vi "Main.vi"() -> ()   [LabVIEW 2014, in "Main Libraryv2.lvlib"]
uses:
  Control/Main Libraryv2.lvlib
  Master/Masterv2.lvclass
  Global/Recipe downloadv2.vi
  Global/Clockwise.Reverse Global.vi
  Global/Admin Enable Globalv2.vi
  Global/User Enablev2.vi
panel:
  in  "Login":bool
  out "Elapsed Time (s)":dbl
  out "Time has Elapsed":bool
  out "error out":errorcluster
  in  "error in (no error)":errorcluster
  out "User Enable":bool
  out "Admin Enable":bool
  in  "Log Out":bool
  in  "Tab Control 2":T1(tab)
  out "Direction":string
  out "Time Limit 2":string
  out "Temperature Limit 2":string
  out "Speed 2":string
  out "Timer":u16
  out "Current Temperature":u16
  in  "Delete":bool
  in  "Add":bool
  in  "Password List":i32(listbox)
  in  "New Password":string
  in  "Recipe Download":u16
  in  "Speed":u16
  in  "Time Limit":u16
  in  "Temperature Limit":u16
  in  "Delete Row":u16
  in  "Recipe":i32(listbox)
  in  "Delete Recipe":bool
  in  "Add Recipe":bool
  in  "Clockwise/Reverse":bool
  in  "Password List 2":i32(listbox)
  in  "Admin Password":string
  in  "Add Admin":bool
  in  "Delete Admin":bool
  in  "Pre Heat and Dry":bool
  in  "Exit":bool
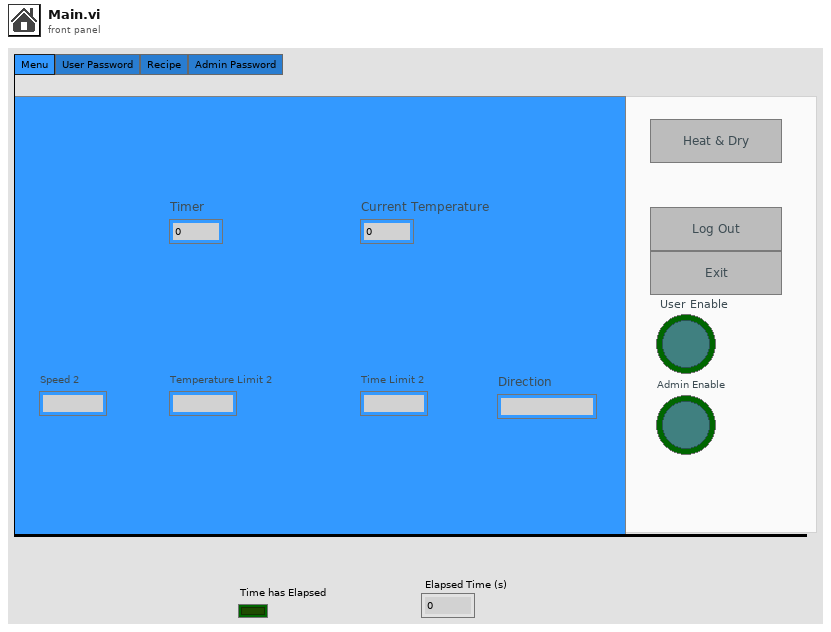
[diagram p1: front panel]
types:
  T1 = enum32{"Menu", "User Password", "Recipe", "Admin Password"}
  T2 = enum16{"9", "8", "7", "6", "5", "4", "3", "2", "1", "0"}[]
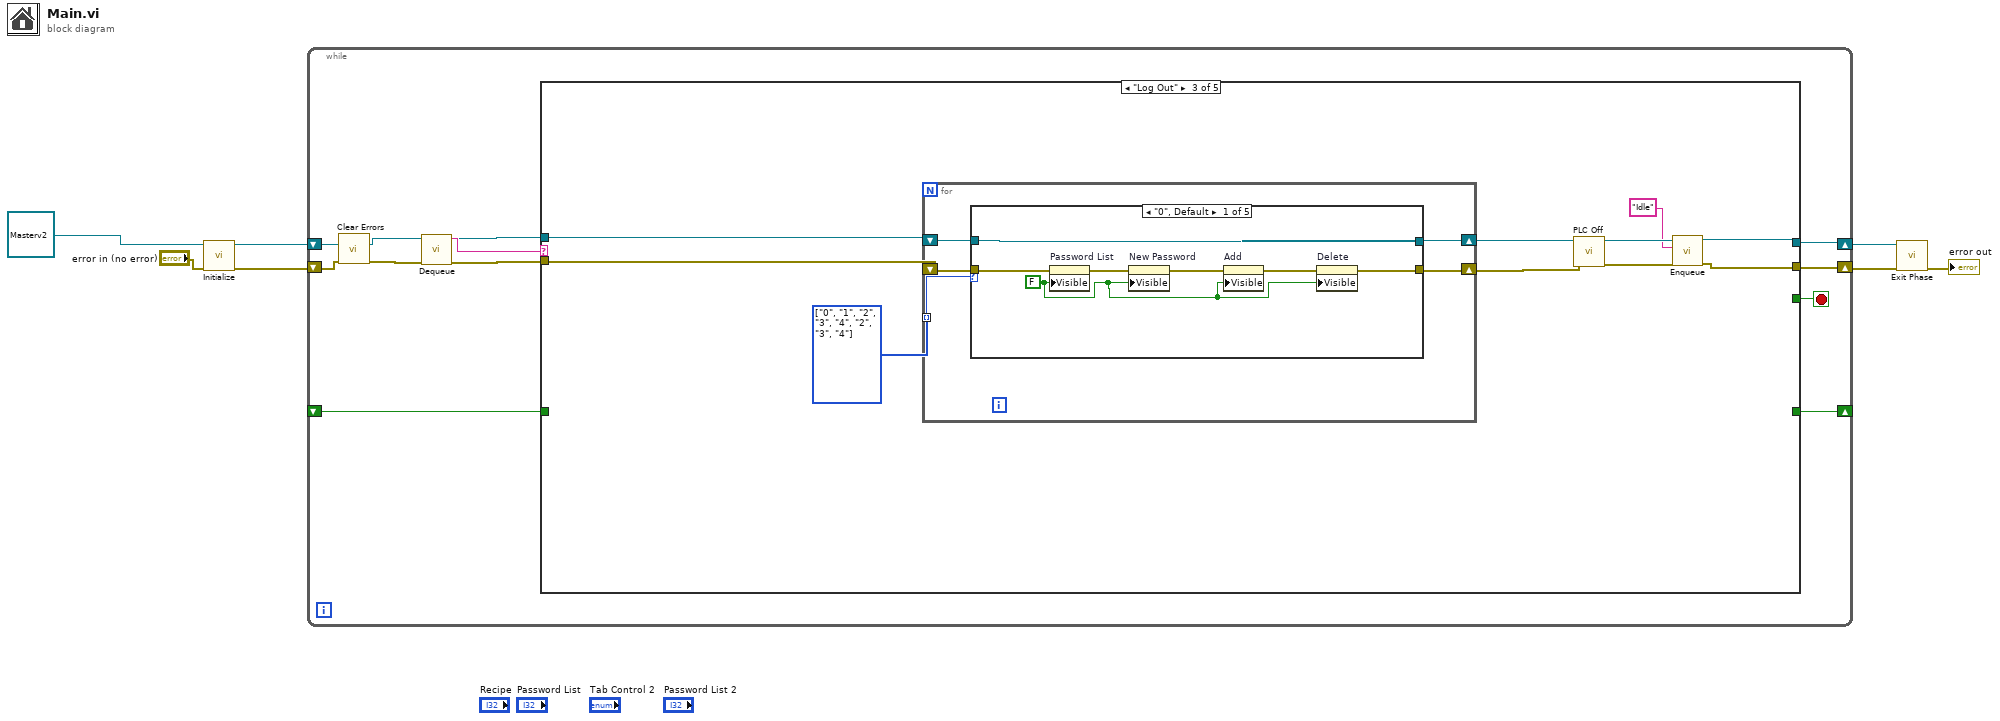
[diagram p0: block diagram]
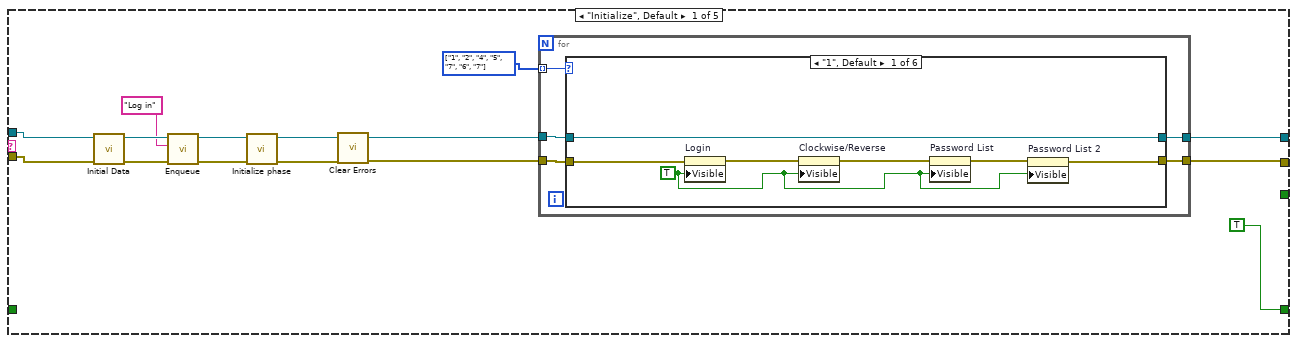
[diagram p2: hidden frame]
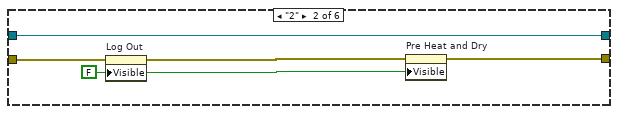
[diagram p3: hidden frame]
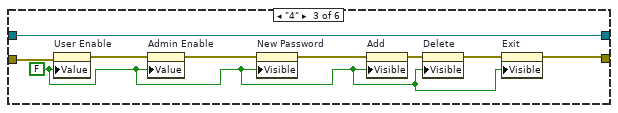
[diagram p4: hidden frame]
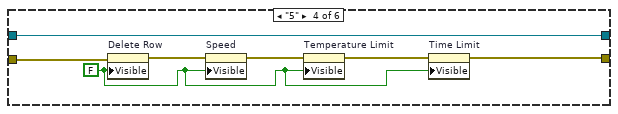
[diagram p5: hidden frame]
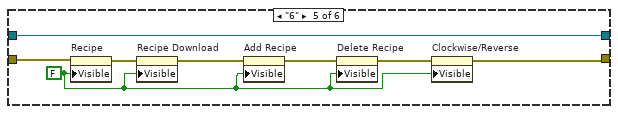
[diagram p6: hidden frame]
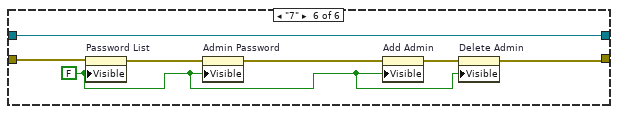
[diagram p7: hidden frame]
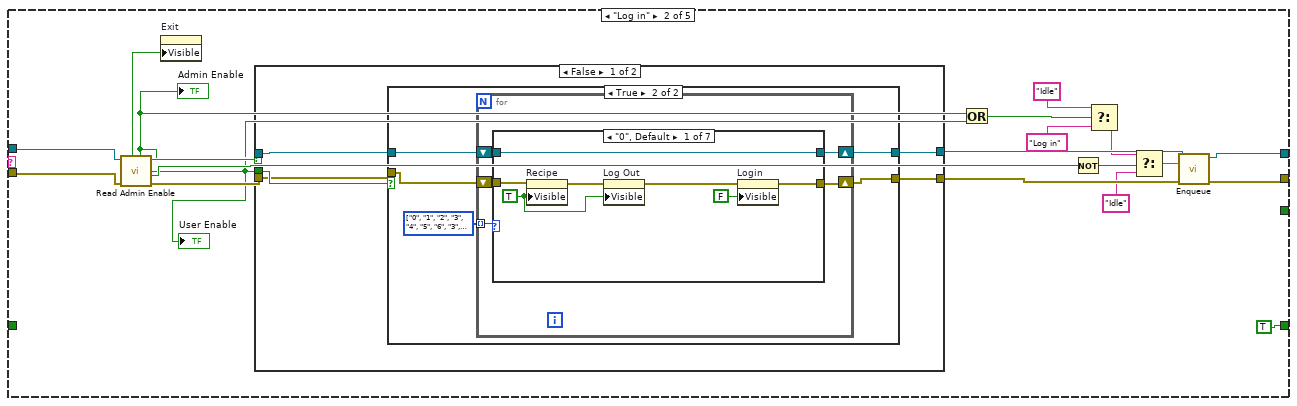
[diagram p8: hidden frame]
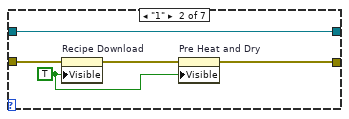
[diagram p10: hidden frame]
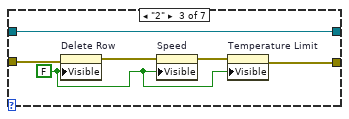
[diagram p11: hidden frame]
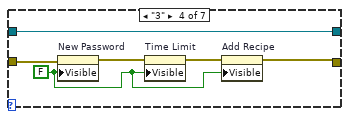
[diagram p12: hidden frame]
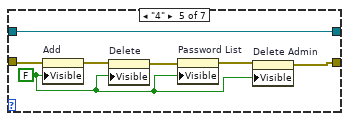
[diagram p13: hidden frame]
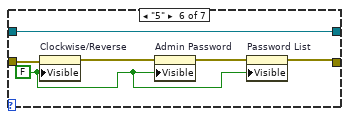
[diagram p14: hidden frame]
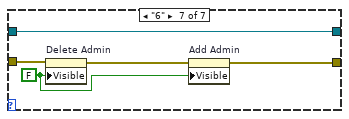
[diagram p15: hidden frame]
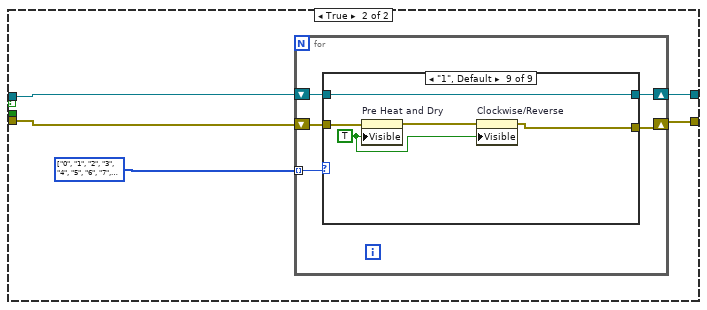
[diagram p16: hidden frame]
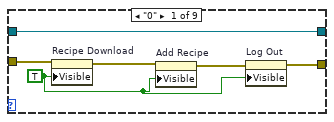
[diagram p17: hidden frame]
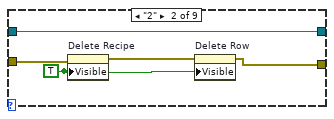
[diagram p18: hidden frame]
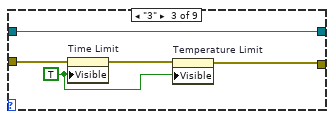
[diagram p19: hidden frame]
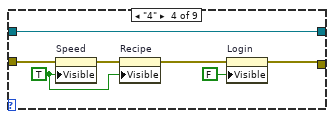
[diagram p20: hidden frame]
diagram:
  n1 = call-dynamic "Initialize.vi"("error in (no error)"="error in (no error)", "Masterv2 in"=refnum<class "Masterv2.lvclass"> refnum ("Main Library.lvlib:Masterv2.lvclass")) -> ("error out"=w4:errorcluster, "Masterv2 out"=w5:refnum<class "Masterv2.lvclass">)  [unwired: 8 in]
  n2 = while {
    shift-right: [w8] -> w2
    shift-left: w4 -> [w18]
    shift-right: [w10] -> w3
    shift-left: w5 -> [w16]
    shift-right: [w12] -> _
    shift-left: _ -> [w11]
    stop <- w9 stop-if-true
    n3 = call <vilib>:"Clear Errors.vi"("error in (no error)"=w18) -> ("error out"=w17:errorcluster)  [unwired: 5 in, 1 out]
    n4 = call-dynamic "Dequeue.vi"("error in (no error)"=w17, "Masterv2 in"=w16) -> ("error out"=w13:errorcluster, "Masterv2 out"=w14:refnum<class "Masterv2.lvclass">, "state"=w15:string)  [unwired: 7 in]
    n5 = case shown="\"Log Out\"" w15 {
      tunnel: w14 -> [w31 w95 w229 w276 w633]
      tunnel: w13 -> [w32 w94 w228 w275 w632]
      tunnel: [TRUE TRUE _ w273 _] -> w12
      tunnel: w11 -> [_ _ _ w274 _]
      tunnel: [w20 w92 w223 w272 w631] -> w10
      tunnel: [w19 w81 w221 w271 w629] -> w8
      tunnel: [_ _ _ _ TRUE] -> w9
      frame "Initialize", Default {
        w23 = enum16{"6", "7", "5", "4", "1", "2"}[] [enum."1", enum."2", enum."4", enum."5", enum."7", enum."6", enum."7"] items=["6", "7", "5", "4", "1", "2"]
        n6 = call-dynamic "Initial Data.vi"("error in (no error)"=w32, "Masterv2 in"=w31) -> ("error out"=w27:errorcluster, "Masterv2 out"=w30:refnum<class "Masterv2.lvclass">)  [unwired: 8 in]
        n7 = call-dynamic "Enqueue.vi"("error in (no error)"=w27, "State"="Log in", "Masterv2 in"=w30) -> ("error out"=w26:errorcluster, "Masterv2 out"=w28:refnum<class "Masterv2.lvclass">)  [unwired: 7 in]
        n8 = call-dynamic "Initialize phase.vi"("error in (no error)"=w26, "Programming Logicv2 in"=w28) -> ("error out"=w25:errorcluster, "Programming Logicv2 out"=w21:refnum<class "Masterv2.lvclass">)  [unwired: 8 in]
        n9 = call <vilib>:"Clear Errors.vi"("error in (no error)"=w25) -> ("error out"=w22:errorcluster)  [unwired: 5 in, 1 out]
        n10 = for {
          tunnel: w23 -> [w37] mode=indexing
          tunnel: w21 -> [w36]
          tunnel: [w35] -> w20
          tunnel: w22 -> [w34]
          tunnel: [w33] -> w19
          n11 = case shown="\"1\", Default" w37 {
            tunnel: w36 -> [w44 w49 w58 w65 w73 w80]
            tunnel: [w44 w49 w58 w65 w73 w80] -> w35
            tunnel: w34 -> [w43 w48 w57 w64 w72 w79]
            tunnel: [w38 w46 w51 w60 w67 w75] -> w33
            frame "1", Default {
              w39 = TRUE ("Visible")
              n12 = property on="Login" class="Bool"(error in=w43, "Visible"=w39) -> (error out=w42:errorcluster)  [unwired: 1 in, 1 out]
              n13 = property on="Clockwise/Reverse" class="Bool (strict)"(error in=w42, "Visible"=w39) -> (error out=w41:errorcluster)  [unwired: 1 in, 1 out]
              n14 = property on="Password List" class="LstBox (strict)"(error in=w41, "Visible"=w39) -> (error out=w40:errorcluster)  [unwired: 1 in, 1 out]
              n15 = property on="Password List 2" class="LstBox (strict)"(error in=w40, "Visible"=w39) -> (error out=w38:errorcluster)  [unwired: 1 in, 1 out]
            }
            frame "2" {
              w45 = FALSE ("Visible")
              n16 = property on="Log Out" class="Bool (strict)"(error in=w48, "Visible"=w45) -> (error out=w47:errorcluster)  [unwired: 1 in, 1 out]
              n17 = property on="Pre Heat and Dry" class="Bool (strict)"(error in=w47, "Visible"=w45) -> (error out=w46:errorcluster)  [unwired: 1 in, 1 out]
            }
            frame "4" {
              w50 = FALSE ("User Enable")
              n18 = property on="User Enable" class="Bool (strict)"(error in=w57, "Value"=w50) -> (error out=w56:errorcluster)  [unwired: 1 in, 1 out]
              n19 = property on="Admin Enable" class="Bool (strict)"(error in=w56, "Value"=w50) -> (error out=w55:errorcluster)  [unwired: 1 in, 1 out]
              n20 = property on="New Password" class="Str"(error in=w55, "Visible"=w50) -> (error out=w54:errorcluster)  [unwired: 1 in, 1 out]
              n21 = property on="Add" class="Bool"(error in=w54, "Visible"=w50) -> (error out=w53:errorcluster)  [unwired: 1 in, 1 out]
              n22 = property on="Delete" class="Bool"(error in=w53, "Visible"=w50) -> (error out=w52:errorcluster)  [unwired: 1 in, 1 out]
              n23 = property on="Exit" class="Bool"(error in=w52, "Visible"=w50) -> (error out=w51:errorcluster)  [unwired: 1 in, 1 out]
            }
            frame "5" {
              w59 = FALSE ("Visible")
              n24 = property on="Delete Row" class="DigNum (strict)"(error in=w64, "Visible"=w59) -> (error out=w63:errorcluster)  [unwired: 1 in, 1 out]
              n25 = property on="Speed" class="DigNum (strict)"(error in=w63, "Visible"=w59) -> (error out=w62:errorcluster)  [unwired: 1 in, 1 out]
              n26 = property on="Temperature Limit" class="DigNum (strict)"(error in=w62, "Visible"=w59) -> (error out=w61:errorcluster)  [unwired: 1 in, 1 out]
              n27 = property on="Time Limit" class="DigNum (strict)"(error in=w61, "Visible"=w59) -> (error out=w60:errorcluster)  [unwired: 1 in, 1 out]
            }
            frame "6" {
              w66 = FALSE ("Visible")
              n28 = property on="Recipe" class="MCListbox (strict)"(error in=w72, "Visible"=w66) -> (error out=w71:errorcluster)  [unwired: 1 in, 1 out]
              n29 = property on="Recipe Download" class="DigNum (strict)"(error in=w71, "Visible"=w66) -> (error out=w70:errorcluster)  [unwired: 1 in, 1 out]
              n30 = property on="Add Recipe" class="Bool"(error in=w70, "Visible"=w66) -> (error out=w69:errorcluster)  [unwired: 1 in, 1 out]
              n31 = property on="Delete Recipe" class="Bool"(error in=w69, "Visible"=w66) -> (error out=w68:errorcluster)  [unwired: 1 in, 1 out]
              n32 = property on="Clockwise/Reverse" class="Bool (strict)"(error in=w68, "Visible"=w66) -> (error out=w67:errorcluster)  [unwired: 1 in, 1 out]
            }
            frame "7" {
              w74 = FALSE ("Visible")
              n33 = property on="Password List" class="LstBox (strict)"(error in=w79, "Visible"=w74) -> (error out=w78:errorcluster)  [unwired: 1 in, 1 out]
              n34 = property on="Admin Password" class="Str"(error in=w78, "Visible"=w74) -> (error out=w77:errorcluster)  [unwired: 1 in, 1 out]
              n35 = property on="Add Admin" class="Bool"(error in=w77, "Visible"=w74) -> (error out=w76:errorcluster)  [unwired: 1 in, 1 out]
              n36 = property on="Delete Admin" class="Bool"(error in=w76, "Visible"=w74) -> (error out=w75:errorcluster)  [unwired: 1 in, 1 out]
            }
          }
        }
      }
      frame "Log in" {
        n37 = call-dynamic "Read Admin Enable.vi"("error in (no error)"=w94, "Masterv2 in"=w95) -> ("error out"=w96:errorcluster, "Boolean"=w84:bool, "Masterv2 out"=w97:refnum<class "Masterv2.lvclass">, "Admin Enable"=w83:bool, "User Enable"=w82:bool, "Programmer Enable"=w93:bool)  [unwired: 4 in]
        "Admin Enable" <- w83
        "User Enable" <- w82
        n38 = property on="Exit" class="Bool"("Visible"=w93) -> ()  [unwired: 2 in, 2 out]
        n39 = case shown="False" w83 {
          tunnel: w82 -> [w105 _]
          tunnel: w96 -> [w103 w164]
          tunnel: w97 -> [w104 w162]
          tunnel: [w101 w163] -> w98
          tunnel: [w102 w161] -> w99
          frame False {
            n40 = case shown="True" w105 {
              tunnel: w104 -> [w107 w112]
              tunnel: w103 -> [w106 w111]
              tunnel: [w107 w110] -> w102
              tunnel: [w106 w109] -> w101
              frame False {
              }
              frame True {
                w108 = enum16{"6", "5", "4", "3", "2", "1", "0"}[] [enum."0", enum."1", enum."2", enum."3", enum."4", enum."5", enum."6", enum."3", enum."4", enum."5", enum."6"] items=["6", "5", "4", "3", "2", "1", "0"]
                n41 = for {
                  shift-right: [w115] -> w110
                  shift-left: w112 -> [w116]
                  shift-right: [w113] -> w109
                  shift-left: w111 -> [w117]
                  tunnel: w108 -> [w114] mode=indexing
                  n42 = case shown="\"0\", Default" w114 {
                    tunnel: w117 -> [w123 w128 w134 w140 w145 w153 w158]
                    tunnel: w116 -> [w124 w129 w135 w141 w148 w154 w159]
                    tunnel: [w124 w129 w135 w141 w148 w154 w159] -> w115
                    tunnel: [w120 w126 w131 w137 w143 w150 w156] -> w113
                    frame "0", Default {
                      w119 = TRUE ("Visible")
                      n43 = property on="Recipe" class="MCListbox (strict)"(error in=w123, "Visible"=w119) -> (error out=w122:errorcluster)  [unwired: 1 in, 1 out]
                      n44 = property on="Log Out" class="Bool (strict)"(error in=w122, "Visible"=w119) -> (error out=w121:errorcluster)  [unwired: 1 in, 1 out]
                      n45 = property on="Login" class="Bool"(error in=w121, "Visible"=FALSE) -> (error out=w120:errorcluster)  [unwired: 1 in, 1 out]
                    }
                    frame "1" {
                      w125 = TRUE ("Visible")
                      n46 = property on="Recipe Download" class="DigNum (strict)"(error in=w128, "Visible"=w125) -> (error out=w127:errorcluster)  [unwired: 1 in, 1 out]
                      n47 = property on="Pre Heat and Dry" class="Bool (strict)"(error in=w127, "Visible"=w125) -> (error out=w126:errorcluster)  [unwired: 1 in, 1 out]
                    }
                    frame "2" {
                      w130 = FALSE ("Visible")
                      n48 = property on="Delete Row" class="DigNum (strict)"(error in=w134, "Visible"=w130) -> (error out=w133:errorcluster)  [unwired: 1 in, 1 out]
                      n49 = property on="Speed" class="DigNum (strict)"(error in=w133, "Visible"=w130) -> (error out=w132:errorcluster)  [unwired: 1 in, 1 out]
                      n50 = property on="Temperature Limit" class="DigNum (strict)"(error in=w132, "Visible"=w130) -> (error out=w131:errorcluster)  [unwired: 1 in, 1 out]
                    }
                    frame "3" {
                      w136 = FALSE ("Visible")
                      n51 = property on="New Password" class="Str"(error in=w140, "Visible"=w136) -> (error out=w139:errorcluster)  [unwired: 1 in, 1 out]
                      n52 = property on="Time Limit" class="DigNum (strict)"(error in=w139, "Visible"=w136) -> (error out=w138:errorcluster)  [unwired: 1 in, 1 out]
                      n53 = property on="Add Recipe" class="Bool"(error in=w138, "Visible"=w136) -> (error out=w137:errorcluster)  [unwired: 1 in, 1 out]
                    }
                    frame "4" {
                      w142 = FALSE ("Visible")
                      n54 = property on="Add" class="Bool"(error in=w145, "Visible"=w142) -> (error out=w146:errorcluster)  [unwired: 1 in, 1 out]
                      n55 = property on="Delete" class="Bool"(error in=w146, "Visible"=w142) -> (error out=w147:errorcluster)  [unwired: 1 in, 1 out]
                      n56 = property on="Password List" class="LstBox (strict)"(error in=w147, "Visible"=w142) -> (error out=w144:errorcluster)  [unwired: 1 in, 1 out]
                      n57 = property on="Delete Admin" class="Bool"(error in=w144, "Visible"=w142) -> (error out=w143:errorcluster)  [unwired: 1 in, 1 out]
                    }
                    frame "5" {
                      w149 = FALSE ("Visible")
                      n58 = property on="Clockwise/Reverse" class="Bool (strict)"(error in=w153, "Visible"=w149) -> (error out=w152:errorcluster)  [unwired: 1 in, 1 out]
                      n59 = property on="Admin Password" class="Str"(error in=w152, "Visible"=w149) -> (error out=w151:errorcluster)  [unwired: 1 in, 1 out]
                      n60 = property on="Password List" class="LstBox (strict)"(error in=w151, "Visible"=w149) -> (error out=w150:errorcluster)  [unwired: 1 in, 1 out]
                    }
                    frame "6" {
                      w155 = FALSE ("Visible")
                      n61 = property on="Delete Admin" class="Bool"(error in=w158, "Visible"=w155) -> (error out=w157:errorcluster)  [unwired: 1 in, 1 out]
                      n62 = property on="Add Admin" class="Bool"(error in=w157, "Visible"=w155) -> (error out=w156:errorcluster)  [unwired: 1 in, 1 out]
                    }
                  }
                }
              }
            }
          }
          frame True {
            w160 = T2 [enum."0", enum."1", enum."2", enum."3", enum."4", enum."5", enum."6", enum."7", enum."8", enum."9"] items=["9", "8", "7", "6", "5", "4", "3", "2", "1", "0"]
            n63 = for {
              shift-right: [w167] -> w161
              shift-left: w162 -> [w168]
              shift-right: [w165] -> w163
              shift-left: w164 -> [w169]
              tunnel: w160 -> [w166] mode=indexing
              n64 = case shown="\"1\", Default" w166 {
                tunnel: w169 -> [w174 w179 w184 w191 w197 w202 w207 w214 w219]
                tunnel: w168 -> [w175 w180 w185 w192 w198 w203 w208 w215 w220]
                tunnel: [w175 w180 w185 w192 w198 w203 w208 w215 w220] -> w167
                tunnel: [w171 w177 w182 w188 w193 w200 w205 w211 w217] -> w165
                frame "0" {
                  w170 = TRUE ("Visible")
                  n65 = property on="Recipe Download" class="DigNum (strict)"(error in=w174, "Visible"=w170) -> (error out=w173:errorcluster)  [unwired: 1 in, 1 out]
                  n66 = property on="Add Recipe" class="Bool"(error in=w173, "Visible"=w170) -> (error out=w172:errorcluster)  [unwired: 1 in, 1 out]
                  n67 = property on="Log Out" class="Bool (strict)"(error in=w172, "Visible"=w170) -> (error out=w171:errorcluster)  [unwired: 1 in, 1 out]
                }
                frame "2" {
                  w176 = TRUE ("Visible")
                  n68 = property on="Delete Recipe" class="Bool"(error in=w179, "Visible"=w176) -> (error out=w178:errorcluster)  [unwired: 1 in, 1 out]
                  n69 = property on="Delete Row" class="DigNum (strict)"(error in=w178, "Visible"=w176) -> (error out=w177:errorcluster)  [unwired: 1 in, 1 out]
                }
                frame "3" {
                  w181 = TRUE ("Visible")
                  n70 = property on="Time Limit" class="DigNum (strict)"(error in=w184, "Visible"=w181) -> (error out=w183:errorcluster)  [unwired: 1 in, 1 out]
                  n71 = property on="Temperature Limit" class="DigNum (strict)"(error in=w183, "Visible"=w181) -> (error out=w182:errorcluster)  [unwired: 1 in, 1 out]
                }
                frame "4" {
                  w187 = TRUE ("Visible")
                  n72 = property on="Speed" class="DigNum (strict)"(error in=w191, "Visible"=w187) -> (error out=w190:errorcluster)  [unwired: 1 in, 1 out]
                  n73 = property on="Recipe" class="MCListbox (strict)"(error in=w190, "Visible"=w187) -> (error out=w189:errorcluster)  [unwired: 1 in, 1 out]
                  n74 = property on="Login" class="Bool"(error in=w189, "Visible"=FALSE) -> (error out=w188:errorcluster)  [unwired: 1 in, 1 out]
                }
                frame "5" {
                  w194 = TRUE ("Visible")
                  n75 = property on="New Password" class="Str"(error in=w197, "Visible"=w194) -> (error out=w196:errorcluster)  [unwired: 1 in, 1 out]
                  n76 = property on="Delete" class="Bool"(error in=w196, "Visible"=w194) -> (error out=w195:errorcluster)  [unwired: 1 in, 1 out]
                  n77 = property on="Password List" class="LstBox (strict)"(error in=w195, "Visible"=w194) -> (error out=w193:errorcluster)  [unwired: 1 in, 1 out]
                }
                frame "6" {
                  w199 = TRUE ("Visible")
                  n78 = property on="Add" class="Bool"(error in=w202, "Visible"=w199) -> (error out=w201:errorcluster)  [unwired: 1 in, 1 out]
                  n79 = property on="Delete" class="Bool"(error in=w201, "Visible"=w199) -> (error out=w200:errorcluster)  [unwired: 1 in, 1 out]
                }
                frame "7" {
                  w204 = TRUE ("Visible")
                  n80 = property on="Password List" class="LstBox (strict)"(error in=w207, "Visible"=w204) -> (error out=w206:errorcluster)  [unwired: 1 in, 1 out]
                  n81 = property on="Admin Password" class="Str"(error in=w206, "Visible"=w204) -> (error out=w205:errorcluster)  [unwired: 1 in, 1 out]
                }
                frame "8" {
                  w210 = TRUE ("Visible")
                  n82 = property on="Add Admin" class="Bool"(error in=w214, "Visible"=w210) -> (error out=w213:errorcluster)  [unwired: 1 in, 1 out]
                  n83 = property on="Delete Admin" class="Bool"(error in=w213, "Visible"=w210) -> (error out=w212:errorcluster)  [unwired: 1 in, 1 out]
                  n84 = property on="Login" class="Bool"(error in=w212, "Visible"=FALSE) -> (error out=w211:errorcluster)  [unwired: 1 in, 1 out]
                }
                frame "1", Default {
                  w216 = TRUE ("Visible")
                  n85 = property on="Pre Heat and Dry" class="Bool (strict)"(error in=w219, "Visible"=w216) -> (error out=w218:errorcluster)  [unwired: 1 in, 1 out]
                  n86 = property on="Clockwise/Reverse" class="Bool (strict)"(error in=w218, "Visible"=w216) -> (error out=w217:errorcluster)  [unwired: 1 in, 1 out]
                }
              }
            }
          }
        }
        n87 = Or(x=w83, y=w82) -> (x .or. y?=w89:bool)
        n88 = Not(x=w84) -> (.not. x?=w87:bool)
        n89 = Select(t="Idle", s=w89, f="Log in" ("State")) -> (s? t:f=w88:string)
        n90 = Select(t=w88, s=w87, f="Idle") -> (s? t:f=w85:string)
        n91 = call-dynamic "Enqueue.vi"("error in (no error)"=w98, "State"=w85, "Masterv2 in"=w99) -> ("error out"=w81:errorcluster, "Masterv2 out"=w92:refnum<class "Masterv2.lvclass">)  [unwired: 7 in]
      }
      frame "Log Out" {
        w230 = enum16{"4", "3", "2", "1", "0"}[] [enum."0", enum."1", enum."2", enum."3", enum."4", enum."2", enum."3", enum."4"] items=["4", "3", "2", "1", "0"]
        n92 = for {
          shift-right: [w233] -> w225
          shift-left: w229 -> [w234]
          shift-right: [w231] -> w224
          shift-left: w228 -> [w232]
          tunnel: w230 -> [w235] mode=indexing
          n93 = case shown="\"0\", Default" w235 {
            tunnel: w234 -> [w242 w249 w257 w263 w270]
            tunnel: [w242 w249 w257 w263 w270] -> w233
            tunnel: w232 -> [w241 w248 w256 w262 w269]
            tunnel: [w237 w244 w252 w259 w265] -> w231
            frame "0", Default {
              w236 = FALSE ("Visible")
              n94 = property on="Password List" class="LstBox (strict)"(error in=w241, "Visible"=w236) -> (error out=w240:errorcluster)  [unwired: 1 in, 1 out]
              n95 = property on="New Password" class="Str"(error in=w240, "Visible"=w236) -> (error out=w239:errorcluster)  [unwired: 1 in, 1 out]
              n96 = property on="Add" class="Bool"(error in=w239, "Visible"=w236) -> (error out=w238:errorcluster)  [unwired: 1 in, 1 out]
              n97 = property on="Delete" class="Bool"(error in=w238, "Visible"=w236) -> (error out=w237:errorcluster)  [unwired: 1 in, 1 out]
            }
            frame "1" {
              w243 = FALSE ("Visible")
              n98 = property on="Recipe" class="MCListbox (strict)"(error in=w248, "Visible"=w243) -> (error out=w247:errorcluster)  [unwired: 1 in, 1 out]
              n99 = property on="Recipe Download" class="DigNum (strict)"(error in=w247, "Visible"=w243) -> (error out=w246:errorcluster)  [unwired: 1 in, 1 out]
              n100 = property on="Delete Row" class="DigNum (strict)"(error in=w246, "Visible"=w243) -> (error out=w245:errorcluster)  [unwired: 1 in, 1 out]
              n101 = property on="Log Out" class="Bool (strict)"(error in=w245, "Visible"=w243) -> (error out=w244:errorcluster)  [unwired: 1 in, 1 out]
            }
            frame "2" {
              w250 = FALSE ("Visible")
              n102 = property on="Speed" class="DigNum (strict)"(error in=w256, "Visible"=w250) -> (error out=w255:errorcluster)  [unwired: 1 in, 1 out]
              n103 = property on="Temperature Limit" class="DigNum (strict)"(error in=w255, "Visible"=w250) -> (error out=w254:errorcluster)  [unwired: 1 in, 1 out]
              n104 = property on="Time Limit" class="DigNum (strict)"(error in=w254, "Visible"=w250) -> (error out=w253:errorcluster)  [unwired: 1 in, 1 out]
              n105 = property on="Login" class="Bool"(error in=w253, "Visible"=TRUE) -> (error out=w252:errorcluster)  [unwired: 1 in, 1 out]
            }
            frame "3" {
              w258 = FALSE ("Visible")
              n106 = property on="Add Recipe" class="Bool"(error in=w262, "Visible"=w258) -> (error out=w261:errorcluster)  [unwired: 1 in, 1 out]
              n107 = property on="Delete Recipe" class="Bool"(error in=w261, "Visible"=w258) -> (error out=w260:errorcluster)  [unwired: 1 in, 1 out]
              n108 = property on="Clockwise/Reverse" class="Bool (strict)"(error in=w260, "Visible"=w258) -> (error out=w259:errorcluster)  [unwired: 1 in, 1 out]
            }
            frame "4" {
              w264 = FALSE ("Visible")
              n109 = property on="Password List" class="LstBox (strict)"(error in=w269, "Visible"=w264) -> (error out=w268:errorcluster)  [unwired: 1 in, 1 out]
              n110 = property on="Admin Password" class="Str"(error in=w268, "Visible"=w264) -> (error out=w267:errorcluster)  [unwired: 1 in, 1 out]
              n111 = property on="Add Admin" class="Bool"(error in=w267, "Visible"=w264) -> (error out=w266:errorcluster)  [unwired: 1 in, 1 out]
              n112 = property on="Delete Admin" class="Bool"(error in=w266, "Visible"=w264) -> (error out=w265:errorcluster)  [unwired: 1 in, 1 out]
            }
          }
        }
        n113 = call-dynamic "PLC Off.vi"("error in (no error)"=w224, "Programming Logicv2 in"=w225) -> ("error out"=w226:errorcluster, "Programming Logicv2 out"=w227:refnum<class "Masterv2.lvclass">)  [unwired: 8 in]
        n114 = call-dynamic "Enqueue.vi"("error in (no error)"=w226, "State"="Idle", "Masterv2 in"=w227) -> ("error out"=w221:errorcluster, "Masterv2 out"=w223:refnum<class "Masterv2.lvclass">)  [unwired: 7 in]
      }
      frame "Idle" {
        n115 = event shown="[0] Timeout" {
          selector: _ -> [_ _ _ _ _ _ _ _ _ _ _ _]
          dyn-events: _ -> [_ _ _ _ _ _ _ _ _ _ _ _]
          timeout: 100 -> [_ _ _ _ _ _ _ _ _ _ _ _]
          tunnel: w276 -> [w302 w313 w326 w459 w523 w537 w555 w569 w583 w597 w600 w617]
          tunnel: w275 -> [w301 w312 w327 w458 w522 w536 w554 w568 w582 w596 w604 w616]
          tunnel: w274 -> [w286 _ _ _ _ _ _ _ _ _ _ _]
          tunnel: [FALSE TRUE TRUE TRUE _ _ _ _ _ _ _ _] -> w273
          tunnel: [w283 w317 w330 w463 w513 w527 w545 w559 w573 w587 w610 w624] -> w272
          tunnel: [w282 w318 w329 w462 w512 w526 w544 w558 w572 w586 w609 w623] -> w271
          event Timeout {
            n116 = event-data() -> ()  [unwired: 1 in, 3 out]
            n117 = call-dynamic "Display Information.vi"("error in (no error)"=w301, "Masterv2 in"=w302) -> ("error out"=w294:errorcluster, "Passwords"=w299:string[], "Masterv2 out"=w295:refnum<class "Masterv2.lvclass">, "Recipe Indicator"=w298:string[][], "Passwords 2"=w300:string[])  [unwired: 5 in]
            n118 = property on="Password List 2" class="LstBox (strict)"("Item Names"=w300) -> ()  [unwired: 2 in, 2 out]
            n119 = property on="Password List" class="LstBox (strict)"("Item Names"=w299) -> ()  [unwired: 2 in, 2 out]
            n120 = property on="Recipe" class="MCListbox (strict)"("ItemNames"=w298) -> ()  [unwired: 2 in, 2 out]
            n121 = call-dynamic "Timeout Phase.vi"("error in (no error)"=w294, "Programming Logicv2 in"=w295) -> ("error out"=w293:errorcluster, "Boolean"=w285:bool, "Programming Logicv2 out"=w291:refnum<class "Masterv2.lvclass">, "Timer"=→"Timer":u16, "Temperature"=→"Current Temperature":u16)  [unwired: 5 in]
            n122 = Or(x=w285, y=w286) -> (x .or. y?=w287:bool)
            n123 = call <vilib>:"Clear Errors.vi"("error in (no error)"=w293) -> ("error out"=w292:errorcluster)  [unwired: 5 in, 1 out]
            n124 = call "Elapsed Time"("Time Target (s)"=600.0, "Reset"=w287, "Set Start Time (s)"=0.0) -> ("Elapsed Time (s)"=→"Elapsed Time (s)":dbl, "Time has Elapsed"=w278:bool)  [unwired: 9 in, 6 out]
            "Time has Elapsed" <- w278
            n125 = Select(t="Log Out", s=w278, f="Idle") -> (s? t:f=w279:string)
            n126 = call-dynamic "Enqueue.vi"("error in (no error)"=w292, "State"=w279, "Masterv2 in"=w291) -> ("error out"=w282:errorcluster, "Masterv2 out"=w283:refnum<class "Masterv2.lvclass">)  [unwired: 7 in]
          }
          event "Pre Heat and Dry": Mouse Up {
            n127 = event-data() -> ()  [unwired: 1 in, 8 out]
            n128 = property on="Recipe" class="MCListbox (strict)"() -> ("ItemNames"=w308:string[][])  [unwired: 2 in, 2 out]
            n129 = global write "Recipe downloadv2.vi" "Recipe Download"("Recipe Download") -> ()
            n130 = call-dynamic "Start Phase.vi"("array"=w308, "error in (no error)"=w312, "index (row)"="Recipe Download", "Programming Logicv2 in"=w313) -> ("error out"=w316:errorcluster, "Speed"=→"Speed 2":string, "Direction"=→"Direction":string, "Programming Logicv2 out"=w314:refnum<class "Masterv2.lvclass">, "Temp"=→"Temperature Limit 2":string, "Time"=→"Time Limit 2":string)  [unwired: 2 in]
            n131 = call <vilib>:"Clear Errors.vi"("error in (no error)"=w316) -> ("error out"=w315:errorcluster)  [unwired: 5 in, 1 out]
            n132 = global write "Clockwise.Reverse Global.vi" "Clockwise/Reverse"("Clockwise/Reverse") -> ()
            n133 = call-dynamic "Enqueue.vi"("error in (no error)"=w315, "State"="Idle", "Masterv2 in"=w314) -> ("error out"=w318:errorcluster, "Masterv2 out"=w317:refnum<class "Masterv2.lvclass">)  [unwired: 7 in]
          }
          event "Login": Value Change {
            n134 = event-data() -> ()  [unwired: 1 in, 6 out]
            n135 = call-dynamic "Read Admin Enable.vi"("error in (no error)"=w327, "Masterv2 in"=w326) -> ("error out"=w323:errorcluster, "Masterv2 out"=w324:refnum<class "Masterv2.lvclass">, "Admin Enable"=w321:bool, "User Enable"=w322:bool, "Programmer Enable"=w325:bool)  [unwired: 4 in, 1 out]
            n136 = property on="Exit" class="Bool"("Visible"=w325) -> ()  [unwired: 2 in, 2 out]
            n137 = global write "Admin Enable Globalv2.vi" "Admin Enable"(w321) -> ()
            n138 = global write "User Enablev2.vi" "User Enable"(w322) -> ()
            n139 = case shown="False" w321 {
              tunnel: w322 -> [w336 _]
              tunnel: w323 -> [w334 w397]
              tunnel: w324 -> [w335 w395]
              tunnel: [w332 w396] -> w319
              tunnel: [w333 w394] -> w320
              frame False {
                n140 = case shown="True" w336 {
                  tunnel: w335 -> [w338 w343]
                  tunnel: w334 -> [w337 w342]
                  tunnel: [w338 w341] -> w333
                  tunnel: [w337 w340] -> w332
                  frame False {
                  }
                  frame True {
                    w339 = enum16{"6", "5", "4", "3", "2", "1", "0"}[] [enum."0", enum."1", enum."2", enum."3", enum."4", enum."5", enum."6", enum."3", enum."4", enum."5", enum."6"] items=["6", "5", "4", "3", "2", "1", "0"]
                    n141 = for {
                      shift-right: [w346] -> w341
                      shift-left: w343 -> [w347]
                      shift-right: [w344] -> w340
                      shift-left: w342 -> [w348]
                      tunnel: w339 -> [w345] mode=indexing
                      n142 = case shown="\"6\"" w345 {
                        tunnel: w348 -> [w354 w359 w365 w371 w376 w384 w391]
                        tunnel: w347 -> [w355 w360 w366 w372 w379 w385 w392]
                        tunnel: [w355 w360 w366 w372 w379 w385 w392] -> w346
                        tunnel: [w351 w357 w362 w368 w374 w381 w387] -> w344
                        frame "0", Default {
                          w350 = TRUE ("Visible")
                          n143 = property on="Recipe" class="MCListbox (strict)"(error in=w354, "Visible"=w350) -> (error out=w353:errorcluster)  [unwired: 1 in, 1 out]
                          n144 = property on="Log Out" class="Bool (strict)"(error in=w353, "Visible"=w350) -> (error out=w352:errorcluster)  [unwired: 1 in, 1 out]
                          n145 = property on="Login" class="Bool"(error in=w352, "Visible"=FALSE) -> (error out=w351:errorcluster)  [unwired: 1 in, 1 out]
                        }
                        frame "1" {
                          w356 = TRUE ("Visible")
                          n146 = property on="Recipe Download" class="DigNum (strict)"(error in=w359, "Visible"=w356) -> (error out=w358:errorcluster)  [unwired: 1 in, 1 out]
                          n147 = property on="Pre Heat and Dry" class="Bool (strict)"(error in=w358, "Visible"=w356) -> (error out=w357:errorcluster)  [unwired: 1 in, 1 out]
                        }
                        frame "2" {
                          w361 = FALSE ("Visible")
                          n148 = property on="Delete Row" class="DigNum (strict)"(error in=w365, "Visible"=w361) -> (error out=w364:errorcluster)  [unwired: 1 in, 1 out]
                          n149 = property on="Speed" class="DigNum (strict)"(error in=w364, "Visible"=w361) -> (error out=w363:errorcluster)  [unwired: 1 in, 1 out]
                          n150 = property on="Temperature Limit" class="DigNum (strict)"(error in=w363, "Visible"=w361) -> (error out=w362:errorcluster)  [unwired: 1 in, 1 out]
                        }
                        frame "3" {
                          w367 = FALSE ("Visible")
                          n151 = property on="New Password" class="Str"(error in=w371, "Visible"=w367) -> (error out=w370:errorcluster)  [unwired: 1 in, 1 out]
                          n152 = property on="Time Limit" class="DigNum (strict)"(error in=w370, "Visible"=w367) -> (error out=w369:errorcluster)  [unwired: 1 in, 1 out]
                          n153 = property on="Add Recipe" class="Bool"(error in=w369, "Visible"=w367) -> (error out=w368:errorcluster)  [unwired: 1 in, 1 out]
                        }
                        frame "4" {
                          w373 = FALSE ("Visible")
                          n154 = property on="Add" class="Bool"(error in=w376, "Visible"=w373) -> (error out=w377:errorcluster)  [unwired: 1 in, 1 out]
                          n155 = property on="Delete" class="Bool"(error in=w377, "Visible"=w373) -> (error out=w378:errorcluster)  [unwired: 1 in, 1 out]
                          n156 = property on="Password List" class="LstBox (strict)"(error in=w378, "Visible"=w373) -> (error out=w375:errorcluster)  [unwired: 1 in, 1 out]
                          n157 = property on="Delete Admin" class="Bool"(error in=w375, "Visible"=w373) -> (error out=w374:errorcluster)  [unwired: 1 in, 1 out]
                        }
                        frame "5" {
                          w380 = FALSE ("Visible")
                          n158 = property on="Clockwise/Reverse" class="Bool (strict)"(error in=w384, "Visible"=w380) -> (error out=w383:errorcluster)  [unwired: 1 in, 1 out]
                          n159 = property on="Admin Password" class="Str"(error in=w383, "Visible"=w380) -> (error out=w382:errorcluster)  [unwired: 1 in, 1 out]
                          n160 = property on="Password List" class="LstBox (strict)"(error in=w382, "Visible"=w380) -> (error out=w381:errorcluster)  [unwired: 1 in, 1 out]
                        }
                        frame "6" {
                          w389 = FALSE ("Visible")
                          n161 = property on="Delete Admin" class="Bool"(error in=w391, "Visible"=w389) -> (error out=w390:errorcluster)  [unwired: 1 in, 1 out]
                          n162 = property on="Add Admin" class="Bool"(error in=w390, "Visible"=w389) -> (error out=w388:errorcluster)  [unwired: 1 in, 1 out]
                          n163 = property on="User Enable" class="Bool (strict)"(error in=w388, "Value"=TRUE ("User Enable")) -> (error out=w387:errorcluster)  [unwired: 1 in, 1 out]
                        }
                      }
                    }
                  }
                }
              }
              frame True {
                w393 = T2 [enum."0", enum."1", enum."2", enum."3", enum."4", enum."5", enum."6", enum."7", enum."8", enum."9"] items=["9", "8", "7", "6", "5", "4", "3", "2", "1", "0"]
                n164 = for {
                  shift-right: [w400] -> w394
                  shift-left: w395 -> [w401]
                  shift-right: [w398] -> w396
                  shift-left: w397 -> [w402]
                  tunnel: w393 -> [w399] mode=indexing
                  n165 = case shown="\"1\", Default" w399 {
                    tunnel: w402 -> [w407 w413 w418 w425 w431 w436 w441 w448 w454]
                    tunnel: w401 -> [w408 w414 w419 w426 w432 w437 w442 w449 w455]
                    tunnel: [w408 w414 w419 w426 w432 w437 w442 w449 w455] -> w400
                    tunnel: [w404 w410 w416 w422 w427 w434 w439 w445 w450] -> w398
                    frame "0" {
                      w403 = TRUE ("Visible")
                      n166 = property on="Recipe Download" class="DigNum (strict)"(error in=w407, "Visible"=w403) -> (error out=w406:errorcluster)  [unwired: 1 in, 1 out]
                      n167 = property on="Add Recipe" class="Bool"(error in=w406, "Visible"=w403) -> (error out=w405:errorcluster)  [unwired: 1 in, 1 out]
                      n168 = property on="Log Out" class="Bool (strict)"(error in=w405, "Visible"=w403) -> (error out=w404:errorcluster)  [unwired: 1 in, 1 out]
                    }
                    frame "2" {
                      w409 = TRUE ("Visible")
                      n169 = property on="Delete Recipe" class="Bool"(error in=w413, "Visible"=w409) -> (error out=w412:errorcluster)  [unwired: 1 in, 1 out]
                      n170 = property on="Delete Row" class="DigNum (strict)"(error in=w412, "Visible"=w409) -> (error out=w411:errorcluster)  [unwired: 1 in, 1 out]
                      n171 = property on="Admin Enable" class="Bool (strict)"(error in=w411, "Value"=w409) -> (error out=w410:errorcluster)  [unwired: 1 in, 1 out]
                    }
                    frame "3" {
                      w415 = TRUE ("Visible")
                      n172 = property on="Time Limit" class="DigNum (strict)"(error in=w418, "Visible"=w415) -> (error out=w417:errorcluster)  [unwired: 1 in, 1 out]
                      n173 = property on="Temperature Limit" class="DigNum (strict)"(error in=w417, "Visible"=w415) -> (error out=w416:errorcluster)  [unwired: 1 in, 1 out]
                    }
                    frame "4" {
                      w421 = TRUE ("Visible")
                      n174 = property on="Speed" class="DigNum (strict)"(error in=w425, "Visible"=w421) -> (error out=w424:errorcluster)  [unwired: 1 in, 1 out]
                      n175 = property on="Recipe" class="MCListbox (strict)"(error in=w424, "Visible"=w421) -> (error out=w423:errorcluster)  [unwired: 1 in, 1 out]
                      n176 = property on="Login" class="Bool"(error in=w423, "Visible"=FALSE) -> (error out=w422:errorcluster)  [unwired: 1 in, 1 out]
                    }
                    frame "5" {
                      w428 = TRUE ("Visible")
                      n177 = property on="New Password" class="Str"(error in=w431, "Visible"=w428) -> (error out=w430:errorcluster)  [unwired: 1 in, 1 out]
                      n178 = property on="Delete" class="Bool"(error in=w430, "Visible"=w428) -> (error out=w429:errorcluster)  [unwired: 1 in, 1 out]
                      n179 = property on="Password List" class="LstBox (strict)"(error in=w429, "Visible"=w428) -> (error out=w427:errorcluster)  [unwired: 1 in, 1 out]
                    }
                    frame "6" {
                      w433 = TRUE ("Visible")
                      n180 = property on="Add" class="Bool"(error in=w436, "Visible"=w433) -> (error out=w435:errorcluster)  [unwired: 1 in, 1 out]
                      n181 = property on="Delete" class="Bool"(error in=w435, "Visible"=w433) -> (error out=w434:errorcluster)  [unwired: 1 in, 1 out]
                    }
                    frame "7" {
                      w438 = TRUE ("Visible")
                      n182 = property on="Password List" class="LstBox (strict)"(error in=w441, "Visible"=w438) -> (error out=w440:errorcluster)  [unwired: 1 in, 1 out]
                      n183 = property on="Admin Password" class="Str"(error in=w440, "Visible"=w438) -> (error out=w439:errorcluster)  [unwired: 1 in, 1 out]
                    }
                    frame "8" {
                      w444 = TRUE ("Visible")
                      n184 = property on="Add Admin" class="Bool"(error in=w448, "Visible"=w444) -> (error out=w447:errorcluster)  [unwired: 1 in, 1 out]
                      n185 = property on="Delete Admin" class="Bool"(error in=w447, "Visible"=w444) -> (error out=w446:errorcluster)  [unwired: 1 in, 1 out]
                      n186 = property on="Login" class="Bool"(error in=w446, "Visible"=FALSE) -> (error out=w445:errorcluster)  [unwired: 1 in, 1 out]
                    }
                    frame "1", Default {
                      w451 = TRUE ("Visible")
                      n187 = property on="Pre Heat and Dry" class="Bool (strict)"(error in=w454, "Visible"=w451) -> (error out=w453:errorcluster)  [unwired: 1 in, 1 out]
                      n188 = property on="Clockwise/Reverse" class="Bool (strict)"(error in=w453, "Visible"=w451) -> (error out=w452:errorcluster)  [unwired: 1 in, 1 out]
                      n189 = property on="User Enable" class="Bool (strict)"(error in=w452, "Value"=w451) -> (error out=w450:errorcluster)  [unwired: 1 in, 1 out]
                    }
                  }
                }
              }
            }
            n190 = call-dynamic "Enqueue.vi"("error in (no error)"=w319, "State"="Idle", "Masterv2 in"=w320) -> ("error out"=w329:errorcluster, "Masterv2 out"=w330:refnum<class "Masterv2.lvclass">)  [unwired: 7 in]
          }
          event "Log Out": Mouse Up {
            w460 = enum16{"4", "3", "2", "1", "0"}[] [enum."0", enum."1", enum."2", enum."3", enum."4", enum."2", enum."3", enum."4"] items=["4", "3", "2", "1", "0"]
            n191 = event-data() -> ()  [unwired: 1 in, 8 out]
            n192 = for {
              shift-right: [w469] -> w457
              shift-left: w459 -> [w470]
              shift-right: [w467] -> w456
              shift-left: w458 -> [w468]
              tunnel: w460 -> [w471] mode=indexing
              n193 = case shown="\"3\"" w471 {
                tunnel: w470 -> [w478 w485 w493 w501 w508]
                tunnel: [w478 w485 w493 w501 w508] -> w469
                tunnel: w468 -> [w477 w484 w492 w500 w507]
                tunnel: [w473 w480 w488 w495 w503] -> w467
                frame "0", Default {
                  w472 = FALSE ("Visible")
                  n194 = property on="Password List" class="LstBox (strict)"(error in=w477, "Visible"=w472) -> (error out=w476:errorcluster)  [unwired: 1 in, 1 out]
                  n195 = property on="New Password" class="Str"(error in=w476, "Visible"=w472) -> (error out=w475:errorcluster)  [unwired: 1 in, 1 out]
                  n196 = property on="Add" class="Bool"(error in=w475, "Visible"=w472) -> (error out=w474:errorcluster)  [unwired: 1 in, 1 out]
                  n197 = property on="Delete" class="Bool"(error in=w474, "Visible"=w472) -> (error out=w473:errorcluster)  [unwired: 1 in, 1 out]
                }
                frame "1" {
                  w479 = FALSE ("Visible")
                  n198 = property on="Recipe" class="MCListbox (strict)"(error in=w484, "Visible"=w479) -> (error out=w483:errorcluster)  [unwired: 1 in, 1 out]
                  n199 = property on="Recipe Download" class="DigNum (strict)"(error in=w483, "Visible"=w479) -> (error out=w482:errorcluster)  [unwired: 1 in, 1 out]
                  n200 = property on="Delete Row" class="DigNum (strict)"(error in=w482, "Visible"=w479) -> (error out=w481:errorcluster)  [unwired: 1 in, 1 out]
                  n201 = property on="Log Out" class="Bool (strict)"(error in=w481, "Visible"=w479) -> (error out=w480:errorcluster)  [unwired: 1 in, 1 out]
                }
                frame "2" {
                  w486 = FALSE ("Visible")
                  n202 = property on="Speed" class="DigNum (strict)"(error in=w492, "Visible"=w486) -> (error out=w491:errorcluster)  [unwired: 1 in, 1 out]
                  n203 = property on="Temperature Limit" class="DigNum (strict)"(error in=w491, "Visible"=w486) -> (error out=w490:errorcluster)  [unwired: 1 in, 1 out]
                  n204 = property on="Time Limit" class="DigNum (strict)"(error in=w490, "Visible"=w486) -> (error out=w489:errorcluster)  [unwired: 1 in, 1 out]
                  n205 = property on="Login" class="Bool"(error in=w489, "Visible"=TRUE) -> (error out=w488:errorcluster)  [unwired: 1 in, 1 out]
                }
                frame "3" {
                  w494 = FALSE ("Visible")
                  n206 = property on="Add Recipe" class="Bool"(error in=w500, "Visible"=w494) -> (error out=w499:errorcluster)  [unwired: 1 in, 1 out]
                  n207 = property on="Delete Recipe" class="Bool"(error in=w499, "Visible"=w494) -> (error out=w498:errorcluster)  [unwired: 1 in, 1 out]
                  n208 = property on="Clockwise/Reverse" class="Bool (strict)"(error in=w498, "Visible"=w494) -> (error out=w497:errorcluster)  [unwired: 1 in, 1 out]
                  n209 = property on="User Enable" class="Bool (strict)"(error in=w497, "Value"=w494) -> (error out=w496:errorcluster)  [unwired: 1 in, 1 out]
                  n210 = property on="Admin Enable" class="Bool (strict)"(error in=w496, "Value"=w494) -> (error out=w495:errorcluster)  [unwired: 1 in, 1 out]
                }
                frame "4" {
                  w502 = FALSE ("Visible")
                  n211 = property on="Password List" class="LstBox (strict)"(error in=w507, "Visible"=w502) -> (error out=w506:errorcluster)  [unwired: 1 in, 1 out]
                  n212 = property on="Admin Password" class="Str"(error in=w506, "Visible"=w502) -> (error out=w505:errorcluster)  [unwired: 1 in, 1 out]
                  n213 = property on="Add Admin" class="Bool"(error in=w505, "Visible"=w502) -> (error out=w504:errorcluster)  [unwired: 1 in, 1 out]
                  n214 = property on="Delete Admin" class="Bool"(error in=w504, "Visible"=w502) -> (error out=w503:errorcluster)  [unwired: 1 in, 1 out]
                }
              }
            }
            n215 = call-dynamic "PLC Off.vi"("error in (no error)"=w456, "Programming Logicv2 in"=w457) -> ("error out"=w465:errorcluster, "Programming Logicv2 out"=w466:refnum<class "Masterv2.lvclass">)  [unwired: 8 in]
            n216 = call-dynamic "Enqueue.vi"("error in (no error)"=w465, "State"="Idle", "Masterv2 in"=w466) -> ("error out"=w462:errorcluster, "Masterv2 out"=w463:refnum<class "Masterv2.lvclass">)  [unwired: 7 in]
          }
          event "Add": Value Change {
            n217 = event-data() -> ()  [unwired: 1 in, 6 out]
            n218 = call-dynamic "Add Password.vi"("error in (no error)"=w522, "Write Password"="New Password", "Masterv2 in"=w523) -> ("error out"=w520:errorcluster, "Masterv2 out"=w521:refnum<class "Masterv2.lvclass">)  [unwired: 7 in]
            n219 = call-dynamic "Path.vi"("error in (no error)"=w520, "pathname"="password", "Masterv2 in"=w521) -> ("error out"=w518:errorcluster, "Masterv2 out"=w519:refnum<class "Masterv2.lvclass">)  [unwired: 7 in]
            n220 = call-dynamic "Write Password.vi"("error in (no error)"=w518, "Masterv2 in"=w519) -> ("error out"=w516:errorcluster, "Masterv2 out"=w517:refnum<class "Masterv2.lvclass">)  [unwired: 8 in]
            n221 = call-dynamic "Write Files.vi"("error in (no error)"=w516, "Masterv2 in"=w517) -> ("error out"=w514:errorcluster, "Masterv2 out"=w515:refnum<class "Masterv2.lvclass">)  [unwired: 8 in]
            n222 = call-dynamic "Enqueue.vi"("error in (no error)"=w514, "State"="Idle", "Masterv2 in"=w515) -> ("error out"=w512:errorcluster, "Masterv2 out"=w513:refnum<class "Masterv2.lvclass">)  [unwired: 7 in]
          }
          event "Add Admin": Value Change {
            n223 = event-data() -> ()  [unwired: 1 in, 6 out]
            n224 = call-dynamic "Add Admin Passwordv2.vi"("error in (no error)"=w536, "Write Password"="Admin Password", "Masterv2 in"=w537) -> ("error out"=w534:errorcluster, "Masterv2 out"=w535:refnum<class "Masterv2.lvclass">)  [unwired: 7 in]
            n225 = call-dynamic "Path.vi"("error in (no error)"=w534, "pathname"="Admin Password", "Masterv2 in"=w535) -> ("error out"=w532:errorcluster, "Masterv2 out"=w533:refnum<class "Masterv2.lvclass">)  [unwired: 7 in]
            n226 = call-dynamic "Write Admin Passwordv2.vi"("error in (no error)"=w532, "Masterv2 in"=w533) -> ("error out"=w530:errorcluster, "Masterv2 out"=w531:refnum<class "Masterv2.lvclass">)  [unwired: 8 in]
            n227 = call-dynamic "Write Files.vi"("error in (no error)"=w530, "Masterv2 in"=w531) -> ("error out"=w528:errorcluster, "Masterv2 out"=w529:refnum<class "Masterv2.lvclass">)  [unwired: 8 in]
            n228 = call-dynamic "Enqueue.vi"("error in (no error)"=w528, "State"="Idle", "Masterv2 in"=w529) -> ("error out"=w526:errorcluster, "Masterv2 out"=w527:refnum<class "Masterv2.lvclass">)  [unwired: 7 in]
          }
          event "Add Recipe": Value Change {
            n229 = event-data() -> ()  [unwired: 1 in, 6 out]
            n230 = call-dynamic "Add Recipe.vi"("Speed"="Speed", "Temperature"="Temperature Limit", "error in (no error)"=w554, "Time Limit"="Time Limit", "Masterv2 in"=w555) -> ("error out"=w552:errorcluster, "Masterv2 out"=w553:refnum<class "Masterv2.lvclass">)  [unwired: 5 in]
            n231 = call-dynamic "Path.vi"("error in (no error)"=w552, "pathname"="Dryer Control", "Masterv2 in"=w553) -> ("error out"=w550:errorcluster, "Masterv2 out"=w551:refnum<class "Masterv2.lvclass">)  [unwired: 7 in]
            n232 = call-dynamic "Write Recipe.vi"("error in (no error)"=w550, "Masterv2 in"=w551) -> ("error out"=w548:errorcluster, "Masterv2 out"=w549:refnum<class "Masterv2.lvclass">)  [unwired: 8 in]
            n233 = call-dynamic "Write Files.vi"("error in (no error)"=w548, "Masterv2 in"=w549) -> ("error out"=w546:errorcluster, "Masterv2 out"=w547:refnum<class "Masterv2.lvclass">)  [unwired: 8 in]
            n234 = call-dynamic "Enqueue.vi"("error in (no error)"=w546, "State"="Idle", "Masterv2 in"=w547) -> ("error out"=w544:errorcluster, "Masterv2 out"=w545:refnum<class "Masterv2.lvclass">)  [unwired: 7 in]
          }
          event "Delete": Value Change {
            n235 = event-data() -> ()  [unwired: 1 in, 6 out]
            n236 = property on="Password List" class="LstBox (strict)"() -> ("Value"=w570:i32)  [unwired: 2 in, 2 out]
            n237 = call-dynamic "Delete Password.vi"("error in (no error)"=w568, "index"=w570, "Masterv2 in"=w569) -> ("error out"=w566:errorcluster, "Masterv2 out"=w567:refnum<class "Masterv2.lvclass">)  [unwired: 7 in]
            n238 = call-dynamic "Path.vi"("error in (no error)"=w566, "pathname"="password", "Masterv2 in"=w567) -> ("error out"=w564:errorcluster, "Masterv2 out"=w565:refnum<class "Masterv2.lvclass">)  [unwired: 7 in]
            n239 = call-dynamic "Write Password.vi"("error in (no error)"=w564, "Masterv2 in"=w565) -> ("error out"=w562:errorcluster, "Masterv2 out"=w563:refnum<class "Masterv2.lvclass">)  [unwired: 8 in]
            n240 = call-dynamic "Write Files.vi"("error in (no error)"=w562, "Masterv2 in"=w563) -> ("error out"=w560:errorcluster, "Masterv2 out"=w561:refnum<class "Masterv2.lvclass">)  [unwired: 8 in]
            n241 = call-dynamic "Enqueue.vi"("error in (no error)"=w560, "State"="Idle", "Masterv2 in"=w561) -> ("error out"=w558:errorcluster, "Masterv2 out"=w559:refnum<class "Masterv2.lvclass">)  [unwired: 7 in]
          }
          event "Delete Admin": Value Change {
            n242 = event-data() -> ()  [unwired: 1 in, 6 out]
            n243 = property on="Password List 2" class="LstBox (strict)"() -> ("Value"=w571:i32)  [unwired: 2 in, 2 out]
            n244 = call-dynamic "Delete Admin Passwordv2.vi"("error in (no error)"=w582, "index"=w571, "Masterv2 in"=w583) -> ("error out"=w580:errorcluster, "Masterv2 out"=w581:refnum<class "Masterv2.lvclass">)  [unwired: 7 in]
            n245 = call-dynamic "Path.vi"("error in (no error)"=w580, "Masterv2 in"=w581) -> ("error out"=w577:errorcluster, "Masterv2 out"=w579:refnum<class "Masterv2.lvclass">)  [unwired: 8 in]
            n246 = call-dynamic "Write Admin Passwordv2.vi"("error in (no error)"=w577, "Masterv2 in"=w579) -> ("error out"=w576:errorcluster, "Masterv2 out"=w578:refnum<class "Masterv2.lvclass">)  [unwired: 8 in]
            n247 = call-dynamic "Write Files.vi"("error in (no error)"=w576, "Masterv2 in"=w578) -> ("error out"=w574:errorcluster, "Masterv2 out"=w575:refnum<class "Masterv2.lvclass">)  [unwired: 8 in]
            n248 = call-dynamic "Enqueue.vi"("error in (no error)"=w574, "State"="Idle", "Masterv2 in"=w575) -> ("error out"=w572:errorcluster, "Masterv2 out"=w573:refnum<class "Masterv2.lvclass">)  [unwired: 7 in]
          }
          event "Delete Recipe": Value Change {
            n249 = event-data() -> ()  [unwired: 1 in, 6 out]
            n250 = call-dynamic "Delete Recipe.vi"("error in (no error)"=w596, "Delete Row"="Delete Row", "Masterv2 in"=w597) -> ("error out"=w594:errorcluster, "Masterv2 out"=w595:refnum<class "Masterv2.lvclass">)  [unwired: 7 in]
            n251 = call-dynamic "Path.vi"("error in (no error)"=w594, "pathname"="Dryer Control", "Masterv2 in"=w595) -> ("error out"=w592:errorcluster, "Masterv2 out"=w593:refnum<class "Masterv2.lvclass">)  [unwired: 7 in]
            n252 = call-dynamic "Write Recipe.vi"("error in (no error)"=w592, "Masterv2 in"=w593) -> ("error out"=w590:errorcluster, "Masterv2 out"=w591:refnum<class "Masterv2.lvclass">)  [unwired: 8 in]
            n253 = call-dynamic "Write Files.vi"("error in (no error)"=w590, "Masterv2 in"=w591) -> ("error out"=w588:errorcluster, "Masterv2 out"=w589:refnum<class "Masterv2.lvclass">)  [unwired: 8 in]
            n254 = call-dynamic "Enqueue.vi"("error in (no error)"=w588, "State"="Idle", "Masterv2 in"=w589) -> ("error out"=w586:errorcluster, "Masterv2 out"=w587:refnum<class "Masterv2.lvclass">)  [unwired: 7 in]
          }
          event "Exit": Value Change {
            w601 = FALSE
            n255 = event-data() -> ()  [unwired: 1 in, 6 out]
            n256 = property on="User Enable" class="Bool (strict)"(error in=w604, "Value"=w601) -> (error out=w603:errorcluster)  [unwired: 1 in, 1 out]
            n257 = property on="Admin Enable" class="Bool (strict)"(error in=w603, "Value"=w601) -> (error out=w602:errorcluster)  [unwired: 1 in, 1 out]
            n258 = call-dynamic "Exit Phase.vi"("error in (no error)"=w602, "Programming Logicv2 in"=w600) -> ("error out"=w606:errorcluster, "Programming Logicv2 out"=w605:refnum<class "Masterv2.lvclass">)  [unwired: 8 in]
            n259 = call <vilib>:"Clear Errors.vi"("error in (no error)"=w606) -> ("error out"=w607:errorcluster)  [unwired: 5 in, 1 out]
            n260 = call-dynamic "Enqueue.vi"("error in (no error)"=w607, "State"="Exit", "Masterv2 in"=w605) -> ("error out"=w609:errorcluster, "Masterv2 out"=w610:refnum<class "Masterv2.lvclass">)  [unwired: 7 in]
          }
          event Panel Close? {
            w613 = FALSE ("Admin Enable")
            n261 = event-data() -> ()  [unwired: 1 in, 4 out]
            n262 = property on="Admin Enable" class="Bool (strict)"(error in=w616, "Value"=w613) -> (error out=w615:errorcluster)  [unwired: 1 in, 1 out]
            n263 = property on="User Enable" class="Bool (strict)"(error in=w615, "Value"=w613) -> (error out=w614:errorcluster)  [unwired: 1 in, 1 out]
            n264 = Two Button Dialog(message="Are you sure you want to close this VI?", 1:"NO" ("F button name (\"Cancel\")"), 2:"YES" ("T button name (\"OK\")")) -> (T button?=w611:bool)
            n265 = call-dynamic "Exit Phase.vi"("error in (no error)"=w614, "Programming Logicv2 in"=w617) -> ("error out"=w618:errorcluster, "Programming Logicv2 out"=w612:refnum<class "Masterv2.lvclass">)  [unwired: 8 in]
            n266 = call <vilib>:"Clear Errors.vi"("error in (no error)"=w618) -> ("error out"=w619:errorcluster)  [unwired: 5 in, 1 out]
            n267 = Select(t="Exit" ("State"), s=w611, f="Idle") -> (s? t:f=w620:string)
            n268 = Not(x=w611) -> (.not. x?=w625:bool)
            n269 = call-dynamic "Enqueue.vi"("error in (no error)"=w619, "State"=w620, "Masterv2 in"=w612) -> ("error out"=w623:errorcluster, "Masterv2 out"=w624:refnum<class "Masterv2.lvclass">)  [unwired: 7 in]
            n270 = event-data("Discard?"=w625) -> ()  [unwired: 1 in, 1 out]
          }
        }
      }
      frame "Exit" {
        n271 = call-dynamic "Release.vi"("error in (no error)"=w632, "Masterv2 in"=w633) -> ("error out"=w629:errorcluster, "Masterv2 out"=w631:refnum<class "Masterv2.lvclass">)  [unwired: 8 in]
      }
    }
  }
  n272 = call-dynamic "Exit Phase.vi"("error in (no error)"=w2, "Programming Logicv2 in"=w3) -> ("error out"=→"error out":errorcluster)  [unwired: 8 in, 1 out]
